vi "Main.vi"(11 "Module Admin":refnum<class "Delacor_lib_QMH_Cloneable Module Admin.lvclass">) -> ()   [LabVIEW 2020, in "Oscilloscope.lvlib"]
doc: "This template is based off of the Queued Message Handler design pattern and the Queued Message Handler project template that ships with LabVIEW.\n\nThe main difference is that the queue is private to this module and communication between modules is performed via Broadcast and Request events.\n\nRequest events are wrapped in public API methods and are handled in the Event Handling Loop (EHL) of this VI. Any module can register for Broadcast events sent by this module. The EHL generates messages based on user interface actions.\n\nThe Message Handling Loop (MHL) processes messages generated by the EHL, or by other messages. The messages are string values, so new messages can be added easily to the Message Cases case structure in the MHL. Each message cluster can also provide an optional value for Message Data, which is a variant that can be converted to whatever message-specific data is required.\n_____\nBased on DQMH Project Template 6.0.0.91."
uses:
  Oscilloscope.lvlib
  <vilib>/Delacor/Delacor QMH/Libraries/Cloneable Module Admin_class/Delacor_lib_QMH_Cloneable Module Admin.lvclass
  C:/Program Files (x86)/National Instruments/LabVIEW 2020/vi.lib/Delacor/Delacor QMH/Libraries/Module Admin_class/Delacor_lib_QMH_Module Admin.lvclass
  Module Data--cluster.ctl
  Clases/Osciloscopio/Osciloscopio.lvclass
  <vilib>/Delacor/Delacor QMH/Libraries/Message Queue_class/Delacor_lib_QMH_Message Queue.lvclass/Delacor_lib_QMH_Message Queue.ctl
  <vilib>/Delacor/Delacor QMH/Libraries/Cloneable Module Admin_class/Delacor_lib_QMH_Cloneable Module Admin.lvclass/Delacor_lib_QMH_Cloneable Module Admin.ctl
  Stop Argument--cluster.ctl
  <vilib>/Delacor/Delacor QMH/Libraries/Module Admin_class/Delacor_lib_QMH_Module Admin.lvclass/Delacor_lib_QMH_Module Admin.ctl
  Set COM Port Argument--cluster.ctl
  Initialize OSC Argument--cluster.ctl
  Close Argument--cluster.ctl
  Autosetup Argument--cluster.ctl
  Configure Channel Argument--cluster.ctl
  Read Waveform Argument--cluster.ctl
  Read Measurement Argument--cluster.ctl
  Read Measurement 2 Channels Argument--cluster.ctl
  Reset Argument--cluster.ctl
  <vilib>/Utility/miscctls.llb/LVPointTypeDef.ctl
  Clases/Osciloscopio/Osciloscopio.lvclass/Osciloscopio.ctl
  <vilib>/Delacor/Delacor QMH/Libraries/Message Queue_class/Delacor_lib_QMH_Enqueue Message (Single).vi
  <vilib>/Delacor/Delacor QMH/Libraries/Cloneable Module Admin_class/Delacor_lib_QMH_Get Module ID.vi
  <vilib>/Delacor/Delacor QMH/Libraries/Module Admin_class/Delacor_lib_QMH_Get External Launch.vi
  Clases/Osciloscopio/Write COM.vi
  <vilib>/Utility/error.llb/Error Cluster From Error Code.vi
  <vilib>/ErrorRing/Error Ring.xnode
  <vilib>/Delacor/Delacor QMH/Libraries/Message Queue_class/Delacor_lib_QMH_Message Queue.lvclass
panel:
  out "error out":errorcluster
  out "Status":string
  in  "Simulate EHL Error":bool
  in  "Simulate MHL Error":bool
  # "Other QMH Modules communicate with this Module via its Public API (wrappers for its Request Events).\n\nThis Module communicates with other Modules via its Broadcast Events.\nAny module that wants to get these messages, just registers for this module's Broadcast events."
  # "This template is for the Delacor Modified Queued Message Handler design pattern.\n\nSee the block diagram for more information on how to use this template."
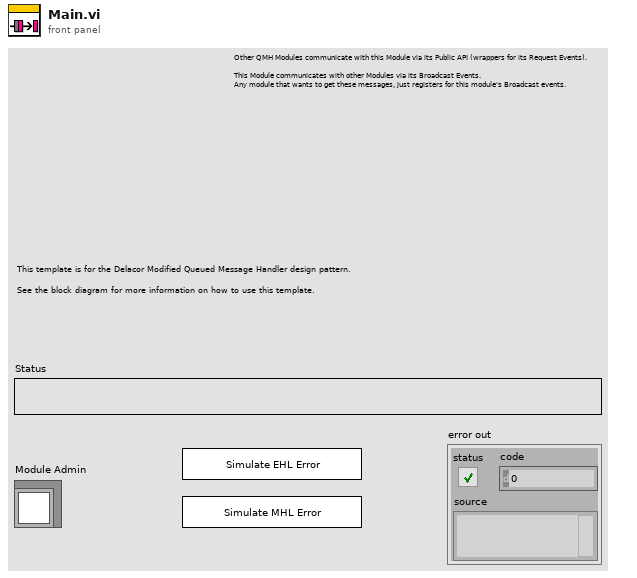
[diagram p1: front panel]
types:
  T1 = typedef "Oscilloscope.lvlib/Request Events--cluster.ctl" = cluster{"Stop Module":refnum<user-event>, "Show Panel":refnum<user-event>, "Hide Panel":refnum<user-event>, "Show Diagram":refnum<user-event>, "Get Module Execution Status":refnum<user-event>, "Set COM Port":refnum<user-event>, "Initialize OSC":refnum<user-event>, "Close":refnum<user-event>, "Autosetup":refnum<user-event>, "Configure Channel":refnum<user-event>, "Read Waveform":refnum<user-event>, "Read Measurement":refnum<user-event>, "Read Measurement 2 Channels":refnum<user-event>, "Reset":refnum<user-event>}
  T2 = typedef "Oscilloscope.lvlib/Module Data--cluster.ctl" = cluster{"Status":string, "Oscilloscope":refnum<class "Osciloscopio.lvclass">}
  T3 = enum32{"invalid lock state", "Not Locked", "Locked (No Password)", "Password-protected"}
  T4 = typedef "Oscilloscope.lvlib/Stop Argument--cluster.ctl" = cluster{"Module ID":i32, "Origin":string, "Exit via Stop Module Req?":bool, "Wait for Module to stop?":bool}
  T5 = typedef "Oscilloscope.lvlib/Set COM Port Argument--cluster.ctl" = cluster{"Module ID":i32, "COM":refnum<visa-resource-name>}
  T6 = typedef "Oscilloscope.lvlib/Initialize OSC Argument--cluster.ctl" = cluster{"Module ID":i32, "OSC Type":string}
  T7 = typedef "Oscilloscope.lvlib/Close Argument--cluster.ctl" = cluster{"Module ID":i32, "Boolean":bool}
  T8 = typedef "Oscilloscope.lvlib/Autosetup Argument--cluster.ctl" = cluster{"Module ID":i32, "Boolean":bool}
  T9 = typedef "Oscilloscope.lvlib/Configure Channel Argument--cluster.ctl" = cluster{"Module ID":i32, "Boolean":bool}
  T10 = typedef "Oscilloscope.lvlib/Read Waveform Argument--cluster.ctl" = cluster{"Module ID":i32, "Boolean":bool}
  T11 = typedef "Oscilloscope.lvlib/Read Measurement Argument--cluster.ctl" = cluster{"Module ID":i32, "Boolean":bool}
  T12 = typedef "Oscilloscope.lvlib/Read Measurement 2 Channels Argument--cluster.ctl" = cluster{"Module ID":i32, "Boolean":bool}
  T13 = typedef "Oscilloscope.lvlib/Reset Argument--cluster.ctl" = cluster{"Module ID":i32, "Boolean":bool}
  T14 = typedef "LVPointTypeDef.ctl" = cluster{"Horizontal":i16, "Vertical":i16}
  T15 = enum32{"Invalid", "Standard", "Closed", "Hidden", "Minimized", "Maximized"}
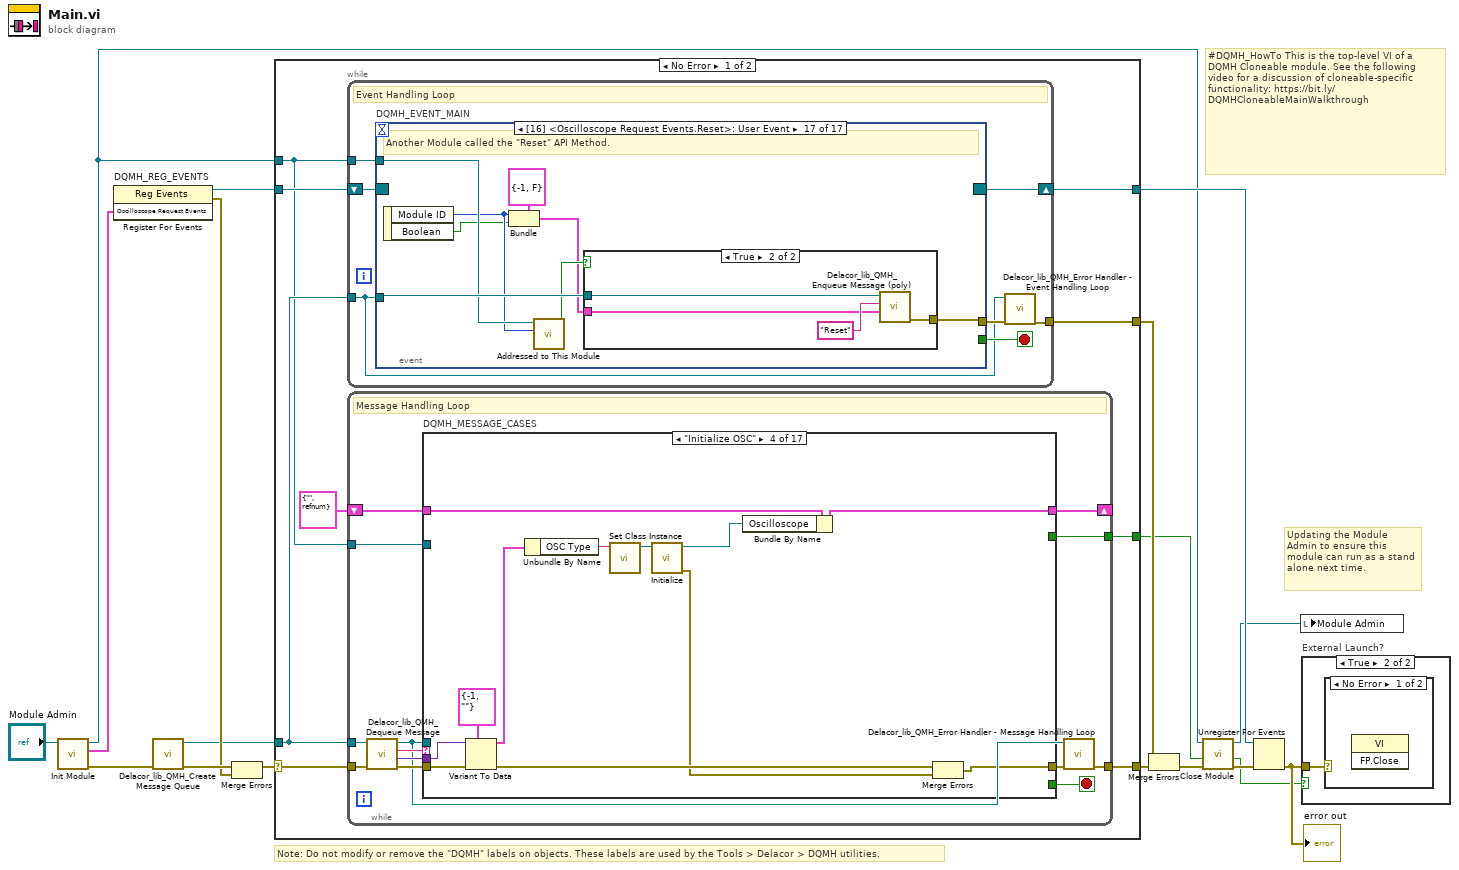
[diagram p0: block diagram]
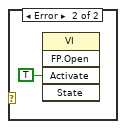
[diagram p3: hidden frame]
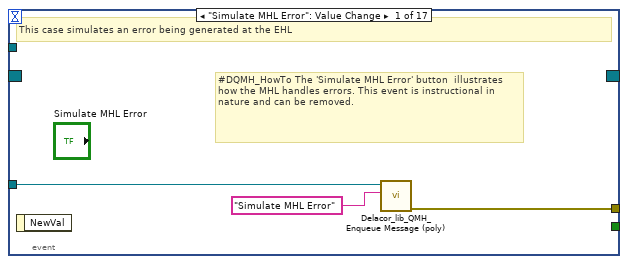
[diagram p4: hidden frame]
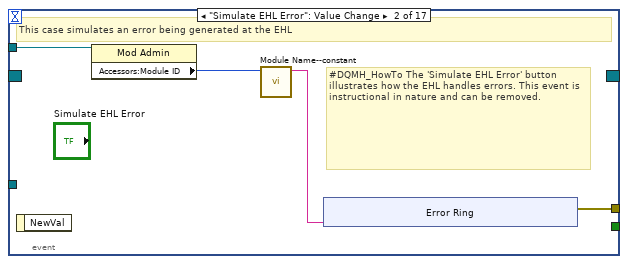
[diagram p5: hidden frame]
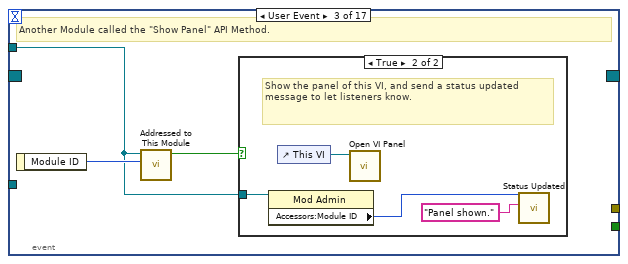
[diagram p6: hidden frame]
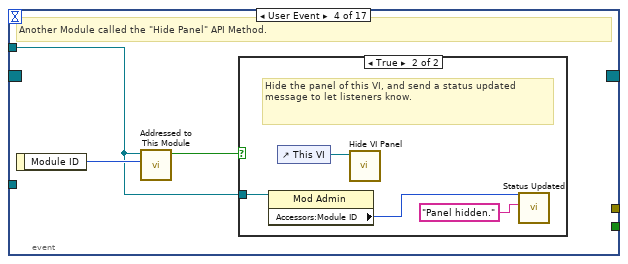
[diagram p8: hidden frame]
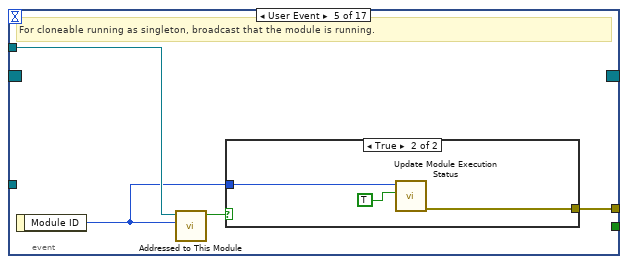
[diagram p10: hidden frame]
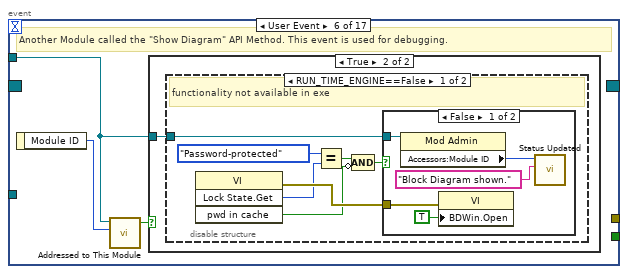
[diagram p12: hidden frame]
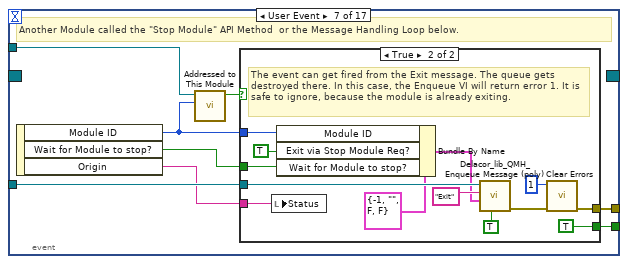
[diagram p16: hidden frame]
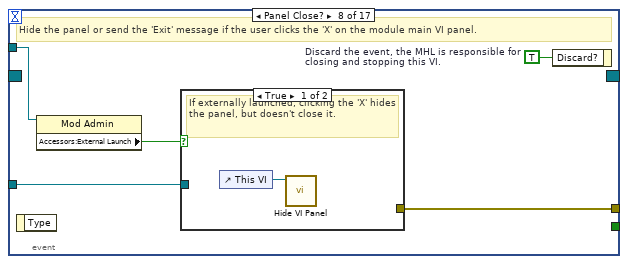
[diagram p18: hidden frame]
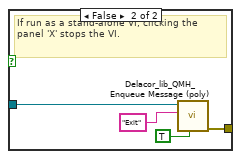
[diagram p19: hidden frame]
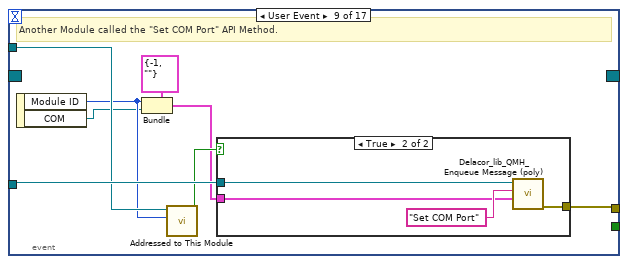
[diagram p20: hidden frame]
diagram:
  # "#DQMH_HowTo This is the top-level VI of a DQMH Cloneable module. See the following video for a discussion of cloneable-specific functionality: https://bit.ly/DQMHCloneableMainWalkthrough"
  # "Note: Do not modify or remove the \"DQMH\" labels on objects. These labels are used by the Tools > Delacor > DQMH utilities."
  # "Updating the Module Admin to ensure this module can run as a stand alone next time."
  n1 = call "Init Module.vi"("Cloneable Module Admin in"="Module Admin") -> ("error out"=w15:errorcluster, "Oscilloscope Request Events"=w7:T1, "Cloneable Module Admin out"=w4:refnum<class "Delacor_lib_QMH_Cloneable Module Admin.lvclass">)  [unwired: 8 in]
  n2 = register-events "DQMH_REG_EVENTS"(w7) -> (reference out=w8:refnum<event-registration>, error out=w10:errorcluster)  [unwired: 2 in]
  n3 = call <vilib>:"Delacor_lib_QMH_Create Message Queue.vi"("error in"=w15) -> ("error out"=w12:errorcluster, "Message Queue"=w6:refnum<class "Delacor_lib_QMH_Message Queue.lvclass">)  [unwired: 9 in]
  n4 = Merge Errors(w12, w10) -> (w11:errorcluster)
  n5 = case shown="No Error" w11 {
    selector: w11 -> [w25 w442]
    tunnel: [w27 w441] -> w16
    tunnel: [w24 w449] -> w9
    tunnel: w8 -> [w22 w449]
    tunnel: w6 -> [w21 w440]
    tunnel: [w26 _] -> w17
    tunnel: w4 -> [w20 w445]
    tunnel: [w19 _] -> w2
    frame No Error {
      n6 = while {
        tunnel: w21 -> [w28]
        shift-right: [w31] -> w24
        shift-left: w22 -> [w32]
        tunnel: [w33] -> w26
        tunnel: w20 -> [w29]
        stop <- w30 stop-if-true
        # "Event Handling Loop"
        n7 = event "DQMH_EVENT_MAIN" shown="[16] <Oscilloscope Request Events.Reset>: User Event" {
          selector: w32 -> [_ _ _ _ _ _ _ _ _ _ _ _ _ _ _ _ _]
          dyn-events: [_ _ _ _ _ _ _ _ _ _ _ _ _ _ _ _ _] -> w31
          timeout: _ -> [_ _ _ _ _ _ _ _ _ _ _ _ _ _ _ _ _]
          tunnel: [_ _ _ _ _ _ w89 _ _ _ _ _ _ _ _ _ _] -> w30
          tunnel: w28 -> [w36 _ _ _ _ _ w92 w108 w124 w136 w148 w160 w172 w184 w196 w208 w220]
          tunnel: [w37 w41 _ _ w66 _ w93 w111 w117 w129 w141 w153 w165 w177 w189 w201 w213] -> w34
          tunnel: w29 -> [_ w40 w49 w56 w64 w70 w91 w109 w122 w134 w146 w158 w170 w182 w194 w206 w218]
          event "Simulate MHL Error": Value Change {
            # "#DQMH_HowTo The 'Simulate MHL Error' button  illustrates how the MHL handles errors. This event is instructional in nature and can be removed."
            # "This case simulates an error being generated at the EHL"
            n8 = event-data() -> ()  [unwired: 1 in, 1 out]
            n9 = call-poly <vilib>:"Delacor_lib_QMH_Enqueue Message (poly).vi"("Message"="Simulate MHL Error", "Message Queue in"=w36) -> ("error out"=w37:errorcluster)  [unwired: 8 in, 1 out]
          }
          event "Simulate EHL Error": Value Change {
            # "#DQMH_HowTo The 'Simulate EHL Error' button  illustrates how the EHL handles errors. This event is instructional in nature and can be removed."
            # "This case simulates an error being generated at the EHL"
            n10 = event-data() -> ()  [unwired: 1 in, 1 out]
            n11 = property class="Mod Admin"(reference=w40) -> ("Accessors:Module ID"=w39:i32)  [unwired: 1 in, 2 out]
            n12 = call "Module Name--constant.vi"("Module ID"=w39) -> ("Module Name"=w38:string)  [unwired: 10 in]
            n13 = xnode "Error Ring"("parameter 0"=w38) -> ("error out"=w41:errorcluster)
          }
          event User Event {
            # "Another Module called the \"Show Panel\" API Method."
            n14 = event-data() -> ("Module ID"=w50:i32)  [unwired: 1 in]
            n15 = call "Addressed to This Module.vi"("Module ID from Argument"=w50, "Module Admin"=w49) -> ("Addressed to this instance?"=w51:bool)  [unwired: 8 in, 1 out]
            n16 = case shown="True" w51 {
              tunnel: w49 -> [_ w53]
              frame False {
              }
              frame True {
                # "Show the panel of this VI, and send a status updated message to let listeners know."
                n17 = property class="Mod Admin"(reference=w53) -> ("Accessors:Module ID"=w52:i32)  [unwired: 1 in, 2 out]
                n18 = control-ref of="This VI"() -> (w55:refnum<vi>)
                n19 = call "Open VI Panel.vi"("VI"=w55) -> ()  [unwired: 10 in, 1 out]
                n20 = call "Status Updated.vi"("Status"="Panel shown." ("format string"), "Module ID"=w52) -> ()  [unwired: 9 in, 1 out]
              }
            }
          }
          event User Event {
            # "Another Module called the \"Hide Panel\" API Method."
            n21 = event-data() -> ("Module ID"=w57:i32)  [unwired: 1 in]
            n22 = call "Addressed to This Module.vi"("Module ID from Argument"=w57, "Module Admin"=w56) -> ("Addressed to this instance?"=w58:bool)  [unwired: 8 in, 1 out]
            n23 = case shown="True" w58 {
              tunnel: w56 -> [_ w60]
              frame False {
              }
              frame True {
                # "Hide the panel of this VI, and send a status updated message to let listeners know."
                n24 = property class="Mod Admin"(reference=w60) -> ("Accessors:Module ID"=w59:i32)  [unwired: 1 in, 2 out]
                n25 = control-ref of="This VI"() -> (w62:refnum<vi>)
                n26 = call "Hide VI Panel.vi"("VI"=w62) -> ()  [unwired: 10 in, 1 out]
                n27 = call "Status Updated.vi"("Status"="Panel hidden." ("format string"), "Module ID"=w59) -> ()  [unwired: 9 in, 1 out]
              }
            }
          }
          event User Event {
            # "For cloneable running as singleton, broadcast that the module is running."
            n28 = event-data() -> ("Module ID"=w63:i32)  [unwired: 1 in]
            n29 = call "Addressed to This Module.vi"("Module ID from Argument"=w63, "Module Admin"=w64) -> ("Addressed to this instance?"=w65:bool)  [unwired: 8 in, 1 out]
            n30 = case shown="True" w65 {
              tunnel: [_ w69] -> w66
              tunnel: w63 -> [_ w68]
              frame False {
              }
              frame True {
                n31 = call "Update Module Execution Status.vi"("Running?"=TRUE, "Module ID"=w68) -> ("error out"=w69:errorcluster)  [unwired: 9 in]
              }
            }
          }
          event User Event {
            # "Another Module called the \"Show Diagram\" API Method. This event is used for debugging."
            n32 = event-data() -> ("Module ID"=w71:i32)  [unwired: 1 in]
            n33 = call "Addressed to This Module.vi"("Module ID from Argument"=w71, "Module Admin"=w70) -> ("Addressed to this instance?"=w72:bool)  [unwired: 8 in, 1 out]
            n34 = case shown="True" w72 {
              tunnel: w70 -> [_ w73]
              frame False {
              }
              frame True {
                n35 = disable-structure shown="RUN_TIME_ENGINE==False" {
                  disable-tunnel: w73 -> [w74 _]
                  frame condition #0 (active) {
                    # "functionality not available in exe"
                    n36 = invoke class="VI" method="Lock State.Get"() -> (error out=w80:errorcluster, "Get Lock State"=w79:T3, "pwd in cache"=w76:bool)  [unwired: 4 in, 1 out]
                    n37 = Equal?(x=T3."Password-protected", y=w79) -> (x = y?=w77:bool)
                    n38 = Compound Arithmetic op=AND(w77, invert w76) -> (w75:bool)
                    n39 = case shown="False" w75 {
                      tunnel: w80 -> [w85 _]
                      tunnel: w74 -> [w82 _]
                      frame False {
                        n40 = property class="Mod Admin"(reference=w82) -> ("Accessors:Module ID"=w81:i32)  [unwired: 1 in, 2 out]
                        n41 = property class="VI"(error in=w85, "BDWin.Open"=TRUE ("Block Diagram Window:Open")) -> ()  [unwired: 1 in, 2 out]
                        n42 = call "Status Updated.vi"("Status"="Block Diagram shown." ("format string"), "Module ID"=w81) -> ()  [unwired: 9 in, 1 out]
                      }
                      frame True {
                        # "Password-protected VI, and the password is not in the cache. Do not show the diagram."
                      }
                    }
                  }
                  frame condition #1 {
                  }
                }
              }
            }
          }
          event User Event {
            # "Another Module called the \"Stop Module\" API Method  or the Message Handling Loop below."
            n43 = event-data() -> ("Module ID"=w87:i32, "Wait for Module to stop?"=w88:bool, "Origin"=w86:string)  [unwired: 1 in]
            n44 = call "Addressed to This Module.vi"("Module ID from Argument"=w87, "Module Admin"=w91) -> ("Addressed to this instance?"=w90:bool)  [unwired: 8 in, 1 out]
            n45 = case shown="True" w90 {
              tunnel: [_ w105] -> w93
              tunnel: w92 -> [_ w101]
              tunnel: [_ TRUE] -> w89
              tunnel: w88 -> [_ w96]
              tunnel: w87 -> [_ w98]
              tunnel: w86 -> [_ w94]
              frame False {
              }
              frame True {
                # "The event can get fired from the Exit message. The queue gets destroyed there. In this case, the Enqueue VI will return error 1. It is safe to ignore, because the module is already exiting."
                n46 = local write "Status"(w94) -> ()
                n47 = Bundle By Name(cluster=T4 {"Module ID"=-1, "Origin"="", "Exit via Stop Module Req?"=FALSE, "Wait for Module to stop?"=FALSE} ("Stop Argument"), "Module ID"=w98, "Exit via Stop Module Req?"=TRUE, "Wait for Module to stop?"=w96) -> (w95:T4)
                n48 = call-poly <vilib>:"Delacor_lib_QMH_Enqueue Message (poly).vi"("Priority Message? (F)"=TRUE, "Message Data"=w95, "Message"="Exit", "Message Queue in"=w101) -> ("error out"=w106:errorcluster)  [unwired: 6 in, 1 out]
                n49 = call <vilib>:"Clear Errors.vi"("error in (no error)"=w106, "specific error code to clear (0: all)"=1) -> ("error out"=w105:errorcluster)  [unwired: 4 in, 1 out]
              }
            }
          }
          event Panel Close? {
            w110 = TRUE  # Discard the event, the MHL is responsible for closing and stopping this VI.
            # "Hide the panel or send the 'Exit' message if the user clicks the 'X' on the module main VI panel."
            n50 = event-data() -> ()  [unwired: 1 in, 1 out]
            n51 = property class="Mod Admin"(reference=w109) -> ("Accessors:External Launch"=w107:bool)  [unwired: 1 in, 2 out]
            n52 = case shown="True" w107 {
              tunnel: w108 -> [_ w115]
              tunnel: [_ w116] -> w111
              frame True {
                # "If externally launched, clicking the 'X' hides the panel, but doesn't close it."
                n53 = control-ref of="This VI"() -> (w112:refnum<vi>)
                n54 = call "Hide VI Panel.vi"("VI"=w112) -> ()  [unwired: 10 in, 1 out]
              }
              frame False {
                # "If run as a stand-alone VI, clicking the panel 'X' stops the VI."
                n55 = call-poly <vilib>:"Delacor_lib_QMH_Enqueue Message (poly).vi"("Priority Message? (F)"=TRUE, "Message"="Exit", "Message Queue in"=w115) -> ("error out"=w116:errorcluster)  [unwired: 7 in, 1 out]
              }
            }
            n56 = event-data("Discard?"=w110) -> ()  [unwired: 1 in, 1 out]
          }
          event User Event {
            # "Another Module called the \"Set COM Port\" API Method."
            n57 = event-data() -> ("Module ID"=w119:i32, "COM"=w118:refnum<visa-resource-name>)  [unwired: 1 in]
            n58 = Bundle(cluster=T5 {"Module ID"=-1, "COM"=""} ("Set COM Port Argument"), "Module ID"=w119, "COM"=w118) -> (w120:T5)
            n59 = call "Addressed to This Module.vi"("Module ID from Argument"=w119, "Module Admin"=w122) -> ("Addressed to this instance?"=w123:bool)  [unwired: 8 in, 1 out]
            n60 = case shown="True" w123 {
              tunnel: w124 -> [_ w128]
              tunnel: w120 -> [_ w126]
              tunnel: [_ w125] -> w117
              frame False {
              }
              frame True {
                n61 = call-poly <vilib>:"Delacor_lib_QMH_Enqueue Message (poly).vi"("Message Data"=w126, "Message"="Set COM Port", "Message Queue in"=w128) -> ("error out"=w125:errorcluster)  [unwired: 7 in, 1 out]
              }
            }
          }
          event User Event {
            # "Another Module called the \"Initialize OSC\" API Method."
            n62 = event-data() -> ("Module ID"=w131:i32, "OSC Type"=w130:string)  [unwired: 1 in]
            n63 = Bundle(cluster=T6 {"Module ID"=-1, "OSC Type"=""} ("Initialize OSC Argument"), "Module ID"=w131, "OSC Type"=w130) -> (w132:T6)
            n64 = call "Addressed to This Module.vi"("Module ID from Argument"=w131, "Module Admin"=w134) -> ("Addressed to this instance?"=w135:bool)  [unwired: 8 in, 1 out]
            n65 = case shown="True" w135 {
              tunnel: w136 -> [_ w140]
              tunnel: w132 -> [_ w138]
              tunnel: [_ w137] -> w129
              frame False {
              }
              frame True {
                n66 = call-poly <vilib>:"Delacor_lib_QMH_Enqueue Message (poly).vi"("Message Data"=w138, "Message"="Initialize OSC", "Message Queue in"=w140) -> ("error out"=w137:errorcluster)  [unwired: 7 in, 1 out]
              }
            }
          }
          event User Event {
            # "Another Module called the \"Close\" API Method."
            n67 = event-data() -> ("Module ID"=w143:i32, "Boolean"=w142:bool)  [unwired: 1 in]
            n68 = Bundle(cluster=T7 {"Module ID"=-1, "Boolean"=FALSE} ("Close Argument"), "Module ID"=w143, "Boolean"=w142) -> (w144:T7)
            n69 = call "Addressed to This Module.vi"("Module ID from Argument"=w143, "Module Admin"=w146) -> ("Addressed to this instance?"=w147:bool)  [unwired: 8 in, 1 out]
            n70 = case shown="True" w147 {
              tunnel: w148 -> [_ w152]
              tunnel: w144 -> [_ w150]
              tunnel: [_ w149] -> w141
              frame False {
              }
              frame True {
                n71 = call-poly <vilib>:"Delacor_lib_QMH_Enqueue Message (poly).vi"("Message Data"=w150, "Message"="Close", "Message Queue in"=w152) -> ("error out"=w149:errorcluster)  [unwired: 7 in, 1 out]
              }
            }
          }
          event User Event {
            # "Another Module called the \"Autosetup\" API Method."
            n72 = event-data() -> ("Module ID"=w155:i32, "Boolean"=w154:bool)  [unwired: 1 in]
            n73 = Bundle(cluster=T8 {"Module ID"=-1, "Boolean"=FALSE} ("Autosetup Argument"), "Module ID"=w155, "Boolean"=w154) -> (w156:T8)
            n74 = call "Addressed to This Module.vi"("Module ID from Argument"=w155, "Module Admin"=w158) -> ("Addressed to this instance?"=w159:bool)  [unwired: 8 in, 1 out]
            n75 = case shown="True" w159 {
              tunnel: w160 -> [_ w164]
              tunnel: w156 -> [_ w162]
              tunnel: [_ w161] -> w153
              frame False {
              }
              frame True {
                n76 = call-poly <vilib>:"Delacor_lib_QMH_Enqueue Message (poly).vi"("Message Data"=w162, "Message"="Autosetup", "Message Queue in"=w164) -> ("error out"=w161:errorcluster)  [unwired: 7 in, 1 out]
              }
            }
          }
          event User Event {
            # "Another Module called the \"Configure Channel\" API Method."
            n77 = event-data() -> ("Module ID"=w167:i32, "Boolean"=w166:bool)  [unwired: 1 in]
            n78 = Bundle(cluster=T9 {"Module ID"=-1, "Boolean"=FALSE} ("Configure Channel Argument"), "Module ID"=w167, "Boolean"=w166) -> (w168:T9)
            n79 = call "Addressed to This Module.vi"("Module ID from Argument"=w167, "Module Admin"=w170) -> ("Addressed to this instance?"=w171:bool)  [unwired: 8 in, 1 out]
            n80 = case shown="True" w171 {
              tunnel: w172 -> [_ w176]
              tunnel: w168 -> [_ w174]
              tunnel: [_ w173] -> w165
              frame False {
              }
              frame True {
                n81 = call-poly <vilib>:"Delacor_lib_QMH_Enqueue Message (poly).vi"("Message Data"=w174, "Message"="Configure Channel", "Message Queue in"=w176) -> ("error out"=w173:errorcluster)  [unwired: 7 in, 1 out]
              }
            }
          }
          event User Event {
            # "Another Module called the \"Read Waveform\" API Method."
            n82 = event-data() -> ("Module ID"=w179:i32, "Boolean"=w178:bool)  [unwired: 1 in]
            n83 = Bundle(cluster=T10 {"Module ID"=-1, "Boolean"=FALSE} ("Read Waveform Argument"), "Module ID"=w179, "Boolean"=w178) -> (w180:T10)
            n84 = call "Addressed to This Module.vi"("Module ID from Argument"=w179, "Module Admin"=w182) -> ("Addressed to this instance?"=w183:bool)  [unwired: 8 in, 1 out]
            n85 = case shown="True" w183 {
              tunnel: w184 -> [_ w188]
              tunnel: w180 -> [_ w186]
              tunnel: [_ w185] -> w177
              frame False {
              }
              frame True {
                n86 = call-poly <vilib>:"Delacor_lib_QMH_Enqueue Message (poly).vi"("Message Data"=w186, "Message"="Read Waveform", "Message Queue in"=w188) -> ("error out"=w185:errorcluster)  [unwired: 7 in, 1 out]
              }
            }
          }
          event User Event {
            # "Another Module called the \"Read Measurement\" API Method."
            n87 = event-data() -> ("Module ID"=w191:i32, "Boolean"=w190:bool)  [unwired: 1 in]
            n88 = Bundle(cluster=T11 {"Module ID"=-1, "Boolean"=FALSE} ("Read Measurement Argument"), "Module ID"=w191, "Boolean"=w190) -> (w192:T11)
            n89 = call "Addressed to This Module.vi"("Module ID from Argument"=w191, "Module Admin"=w194) -> ("Addressed to this instance?"=w195:bool)  [unwired: 8 in, 1 out]
            n90 = case shown="True" w195 {
              tunnel: w196 -> [_ w200]
              tunnel: w192 -> [_ w198]
              tunnel: [_ w197] -> w189
              frame False {
              }
              frame True {
                n91 = call-poly <vilib>:"Delacor_lib_QMH_Enqueue Message (poly).vi"("Message Data"=w198, "Message"="Read Measurement", "Message Queue in"=w200) -> ("error out"=w197:errorcluster)  [unwired: 7 in, 1 out]
              }
            }
          }
          event User Event {
            # "Another Module called the \"Read Measurement 2 Channels\" API Method."
            n92 = event-data() -> ("Module ID"=w203:i32, "Boolean"=w202:bool)  [unwired: 1 in]
            n93 = Bundle(cluster=T12 {"Module ID"=-1, "Boolean"=FALSE} ("Read Measurement 2 Channels Argument"), "Module ID"=w203, "Boolean"=w202) -> (w204:T12)
            n94 = call "Addressed to This Module.vi"("Module ID from Argument"=w203, "Module Admin"=w206) -> ("Addressed to this instance?"=w207:bool)  [unwired: 8 in, 1 out]
            n95 = case shown="True" w207 {
              tunnel: w208 -> [_ w212]
              tunnel: w204 -> [_ w210]
              tunnel: [_ w209] -> w201
              frame False {
              }
              frame True {
                n96 = call-poly <vilib>:"Delacor_lib_QMH_Enqueue Message (poly).vi"("Message Data"=w210, "Message"="Read Measurement 2 Channels", "Message Queue in"=w212) -> ("error out"=w209:errorcluster)  [unwired: 7 in, 1 out]
              }
            }
          }
          event User Event {
            # "Another Module called the \"Reset\" API Method."
            n97 = event-data() -> ("Module ID"=w215:i32, "Boolean"=w214:bool)  [unwired: 1 in]
            n98 = Bundle(cluster=T13 {"Module ID"=-1, "Boolean"=FALSE} ("Reset Argument"), "Module ID"=w215, "Boolean"=w214) -> (w216:T13)
            n99 = call "Addressed to This Module.vi"("Module ID from Argument"=w215, "Module Admin"=w218) -> ("Addressed to this instance?"=w219:bool)  [unwired: 8 in, 1 out]
            n100 = case shown="True" w219 {
              tunnel: w220 -> [_ w224]
              tunnel: w216 -> [_ w222]
              tunnel: [_ w221] -> w213
              frame False {
              }
              frame True {
                n101 = call-poly <vilib>:"Delacor_lib_QMH_Enqueue Message (poly).vi"("Message Data"=w222, "Message"="Reset", "Message Queue in"=w224) -> ("error out"=w221:errorcluster)  [unwired: 7 in, 1 out]
              }
            }
          }
        }
        n102 = call-dynamic "Delacor_lib_QMH_Error Handler - Event Handling Loop.vi"("error in"=w34, "Message Queue in"=w28) -> ("dup error in"=w33:errorcluster)  [unwired: 8 in, 1 out]
      }
      n103 = while {
        tunnel: w21 -> [w228]
        shift-right: [w232] -> _
        shift-left: T2 {"Status"="", "Oscilloscope"=refnum} ("Data Cluster") -> [w233]
        tunnel: w25 -> [w236]
        tunnel: [w234] -> w27
        tunnel: w20 -> [w226]
        tunnel: [w225] -> w19
        stop <- w231 stop-if-true
        # "Message Handling Loop"
        n104 = call-dynamic "Delacor_lib_QMH_Dequeue Message.vi"("error in"=w236, "Message Queue in"=w228) -> ("error out"=w235:errorcluster, "Message Data"=w229:variant, "Message"=w230:string, "Message Queue out"=w227:refnum<class "Delacor_lib_QMH_Message Queue.lvclass">)  [unwired: 6 in]
        n105 = case "DQMH_MESSAGE_CASES" shown="\"Initialize OSC\"" w230 {
          selector: w230 -> [_ _ _ _ _ _ _ _ _ _ _ _ _ _ _ _ w427]
          tunnel: w227 -> [_ _ _ _ _ _ _ _ _ _ _ _ _ w378 _ w417 _]
          tunnel: w235 -> [w257 w261 w271 w287 w296 w308 w320 w332 w344 w356 w368 w374 w376 w387 w400 w423 w429]
          tunnel: [w255 w261 w263 w280 w289 w301 w313 w325 w337 w349 w361 w373 w376 w383 w399 w420 w430] -> w237
          tunnel: w233 -> [w248 w260 w266 w282 w291 w303 w315 w327 w339 w351 w363 w372 w375 w382 w397 w416 w428]
          tunnel: [w247 w260 w265 w281 w290 w302 w314 w326 w338 w350 w362 w372 w375 w382 w397 w416 w428] -> w232
          tunnel: [_ _ _ _ _ _ _ _ _ _ _ _ _ _ _ w415 _] -> w231
          tunnel: w229 -> [_ _ w269 w285 w294 w306 w318 w330 w342 w354 w366 _ _ w381 _ w413 _]
          tunnel: w226 -> [w243 _ _ _ _ _ _ _ _ _ _ _ _ w380 w395 w409 w425]
          tunnel: [_ _ _ _ _ _ _ _ _ _ _ _ _ _ _ w411 _] -> w225
          frame "Initialize" {
            w240 = "Initial Message" ("Initial Message")
            # "Initialize - Any operation that needs to be done before the module can receive messages. Synchronize Caller Events.vi will inform Start Module.vi that the module has launched and is ready to receive messages. Module Did Init.vi will broadcast that the module initialized."
            n106 = call "Synchronize Caller Events.vi"("error in (no error)"=w257, "Module Admin"=w243) -> ("error out"=w256:errorcluster, "Module Admin out"=w242:refnum<class "Delacor_lib_QMH_Cloneable Module Admin.lvclass">)  [unwired: 8 in]
            n107 = call "Get Classes Names.vi"() -> ("Array"=w239:string[])  [unwired: 11 in]
            n108 = property class="Mod Admin"(reference=w242) -> ("Accessors:Module ID"=w238:i32, "Accessors:External Launch"=w244:bool)  [unwired: 1 in, 2 out]
            n109 = call "OSC Availables.vi"("OSC Type"=w239, "Module ID"=w238) -> ()  [unwired: 9 in, 1 out]
            n110 = call "Module Name--constant.vi"("Module ID"=w238) -> ("Module Name"=w252:string)  [unwired: 10 in]
            n111 = property class="VI"("Front Panel.Title"=w252) -> (reference out=w254:refnum<vi>, error out=w259:errorcluster)  [unwired: 2 in]
            n112 = Select(t=T15."Hidden" ("State"), s=w244, f=T15."Standard" ("State")) -> (s? t:f=w249:T15)
            n113 = invoke class="VI" method="FP.Open"(reference=w254, error in=w259, "State"=w249) -> (reference out=w253:refnum<vi>, error out=w258:errorcluster)  [unwired: 2 in, 3 out]
            n114 = call "Module Name--constant.vi"("Module ID"=w238) -> ("Module Name"=w245:string)  [unwired: 10 in]
            n115 = Bundle By Name(cluster=w248, "Status"=w240) -> (w247:T2)
            n116 = invoke class="VI" method="FP.Center"(reference=w253, error in=w258) -> ()  [unwired: 1 in, 3 out]
            n117 = property on="Pane" class="Pane"("Origin"=T14 {"Horizontal"=0, "Vertical"=0}) -> ()  [unwired: 2 in, 2 out]
            n118 = call "Module Did Init.vi"("error in (no error)"=w256, "Initialized?"=TRUE, "Origin"=w245, "Module ID"=w238) -> ("error out"=w255:errorcluster)  [unwired: 7 in]
            "Status" <- w240
          }
          frame "---Module Specific---" {
            # "Separator -- The following cases handle messages specific to this Module."
          }
          frame "Set COM Port" {
            # "Set the COM Port"
            n119 = Variant To Data(error in=w271, type=T5 {"Module ID"=-1, "COM"=""} ("Set COM Port Argument"), Variant=w269) -> (data=w267:T5, error out=w270:errorcluster)
            n120 = Unbundle By Name(w267) -> ("COM"=w264:refnum<visa-resource-name>)
            n121 = in-place {
              in-place-border: w264 -> [w275]
              in-place-border: [w272] -> w262
              n122 = in-place-cluster #1(w266) -> ("Oscilloscope"=w274:refnum<class "Osciloscopio.lvclass">)
              n123 = property class="Osciloscopio.lvclass"(reference=w274, "Accessors:COM"=w275) -> (reference out=w273:refnum<class "Osciloscopio.lvclass">, error out=w272:errorcluster)  [unwired: 1 in]
              n124 = in-place-cluster #1("Oscilloscope"=w273) -> (w265:T2)
            }
            n125 = Merge Errors(w270, w262) -> (w263:errorcluster)
          }
          frame "Initialize OSC" {
            n126 = Variant To Data(error in=w287, type=T6 {"Module ID"=-1, "OSC Type"=""} ("Initialize OSC Argument"), Variant=w285) -> (data=w283:T6, error out=w286:errorcluster)
            n127 = Unbundle By Name(w283) -> ("OSC Type"=w278:string)
            n128 = call "Set Class Instance.vi"("OSC Type"=w278) -> ("element"=w276:refnum<class "Osciloscopio.lvclass">)  [unwired: 10 in]
            n129 = call-dynamic "Initialize.vi"("Osciloscopio in"=w276) -> ("error out"=w279:errorcluster, "Osciloscopio out"=w277:refnum<class "Osciloscopio.lvclass">)  [unwired: 9 in]
            n130 = Bundle By Name(cluster=w282, "Oscilloscope"=w277) -> (w281:T2)
            n131 = Merge Errors(w286, w279) -> (w280:errorcluster)
          }
          frame "Close" {
            # "Close OSC"
            n132 = Variant To Data(error in=w296, type=T7 {"Module ID"=-1, "Boolean"=FALSE} ("Close Argument"), Variant=w294) -> (data=w292:T7, error out=w295:errorcluster)
            n133 = Unbundle By Name(w292) -> ()  [unwired: 2 out]
            n134 = in-place {
              in-place-border: [w297] -> w288
              n135 = in-place-cluster #2(w291) -> ("Oscilloscope"=w299:refnum<class "Osciloscopio.lvclass">)
              n136 = call-dynamic "Close.vi"("Osciloscopio in"=w299) -> ("error out"=w297:errorcluster, "Osciloscopio out"=w298:refnum<class "Osciloscopio.lvclass">)  [unwired: 9 in]
              n137 = in-place-cluster #2("Oscilloscope"=w298) -> (w290:T2)
            }
            n138 = Merge Errors(w295, w288) -> (w289:errorcluster)
          }
          frame "Autosetup" {
            # "Autoset OSC"
            n139 = Variant To Data(error in=w308, type=T8 {"Module ID"=-1, "Boolean"=FALSE} ("Autosetup Argument"), Variant=w306) -> (data=w304:T8, error out=w307:errorcluster)
            n140 = Unbundle By Name(w304) -> ()  [unwired: 2 out]
            n141 = in-place {
              in-place-border: [w309] -> w300
              n142 = in-place-cluster #3(w303) -> ("Oscilloscope"=w311:refnum<class "Osciloscopio.lvclass">)
              n143 = call-dynamic "Autosetup.vi"("Osciloscopio in"=w311) -> ("error out"=w309:errorcluster, "Osciloscopio out"=w310:refnum<class "Osciloscopio.lvclass">)  [unwired: 9 in]
              n144 = in-place-cluster #3("Oscilloscope"=w310) -> (w302:T2)
            }
            n145 = Merge Errors(w307, w300) -> (w301:errorcluster)
          }
          frame "Configure Channel" {
            # "Configure channel of OSC"
            n146 = Variant To Data(error in=w320, type=T9 {"Module ID"=-1, "Boolean"=FALSE} ("Configure Channel Argument"), Variant=w318) -> (data=w316:T9, error out=w319:errorcluster)
            n147 = Unbundle By Name(w316) -> ()  [unwired: 2 out]
            n148 = in-place {
              in-place-border: [w321] -> w312
              n149 = in-place-cluster #4(w315) -> ("Oscilloscope"=w323:refnum<class "Osciloscopio.lvclass">)
              n150 = call-dynamic "Configure Channel.vi"("Osciloscopio in"=w323) -> ("error out"=w321:errorcluster, "Osciloscopio out"=w322:refnum<class "Osciloscopio.lvclass">)  [unwired: 9 in]
              n151 = in-place-cluster #4("Oscilloscope"=w322) -> (w314:T2)
            }
            n152 = Merge Errors(w319, w312) -> (w313:errorcluster)
          }
          frame "Read Waveform" {
            # "Reads the waveform"
            n153 = Variant To Data(error in=w332, type=T10 {"Module ID"=-1, "Boolean"=FALSE} ("Read Waveform Argument"), Variant=w330) -> (data=w328:T10, error out=w331:errorcluster)
            n154 = in-place {
              in-place-border: [w333] -> w324
              n155 = in-place-cluster #5(w327) -> ("Oscilloscope"=w335:refnum<class "Osciloscopio.lvclass">)
              n156 = call-dynamic "Read (Waveform).vi"("Osciloscopio in"=w335) -> ("error out"=w333:errorcluster, "Osciloscopio out"=w334:refnum<class "Osciloscopio.lvclass">)  [unwired: 8 in, 1 out]
              n157 = in-place-cluster #5("Oscilloscope"=w334) -> (w326:T2)
            }
            n158 = Unbundle By Name(w328) -> ()  [unwired: 2 out]
            n159 = Merge Errors(w331, w324) -> (w325:errorcluster)
          }
          frame "Read Measurement" {
            # "Reads the measure"
            n160 = Variant To Data(error in=w344, type=T11 {"Module ID"=-1, "Boolean"=FALSE} ("Read Measurement Argument"), Variant=w342) -> (data=w340:T11, error out=w343:errorcluster)
            n161 = in-place {
              in-place-border: [w345] -> w336
              n162 = in-place-cluster #6(w339) -> ("Oscilloscope"=w347:refnum<class "Osciloscopio.lvclass">)
              n163 = call-dynamic "Read Measurement.vi"("Osciloscopio in"=w347) -> ("error out"=w345:errorcluster, "Osciloscopio out"=w346:refnum<class "Osciloscopio.lvclass">)  [unwired: 7 in, 2 out]
              n164 = in-place-cluster #6("Oscilloscope"=w346) -> (w338:T2)
            }
            n165 = Unbundle By Name(w340) -> ()  [unwired: 2 out]
            n166 = Merge Errors(w343, w336) -> (w337:errorcluster)
          }
          frame "Read Measurement 2 Channels" {
            # "Reads the measure of the 2 Channels of OSC"
            n167 = Variant To Data(error in=w356, type=T12 {"Module ID"=-1, "Boolean"=FALSE} ("Read Measurement 2 Channels Argument"), Variant=w354) -> (data=w352:T12, error out=w355:errorcluster)
            n168 = Unbundle By Name(w352) -> ()  [unwired: 2 out]
            n169 = in-place {
              in-place-border: [w357] -> w348
              n170 = in-place-cluster #7(w351) -> ("Oscilloscope"=w359:refnum<class "Osciloscopio.lvclass">)
              n171 = call-dynamic "Read Measurement 2 Channels.vi"("Osciloscopio in"=w359) -> ("error out"=w357:errorcluster, "Osciloscopio out"=w358:refnum<class "Osciloscopio.lvclass">)  [unwired: 7 in, 2 out]
              n172 = in-place-cluster #7("Oscilloscope"=w358) -> (w350:T2)
            }
            n173 = Merge Errors(w355, w348) -> (w349:errorcluster)
          }
          frame "Reset" {
            # "Resets the OSC"
            n174 = Variant To Data(error in=w368, type=T13 {"Module ID"=-1, "Boolean"=FALSE} ("Reset Argument"), Variant=w366) -> (data=w364:T13, error out=w367:errorcluster)
            n175 = in-place {
              in-place-border: [w369] -> w360
              n176 = in-place-cluster #8(w363) -> ("Oscilloscope"=w370:refnum<class "Osciloscopio.lvclass">)
              n177 = call-dynamic "Reset.vi"("Osciloscopio in"=w370) -> ("error out"=w369:errorcluster, "Osciloscopio out"=w371:refnum<class "Osciloscopio.lvclass">)  [unwired: 9 in]
              n178 = in-place-cluster #8("Oscilloscope"=w371) -> (w362:T2)
            }
            n179 = Unbundle By Name(w364) -> ()  [unwired: 2 out]
            n180 = Merge Errors(w367, w360) -> (w361:errorcluster)
          }
          frame "---Copy This Frame---" {
            # "Duplicate this frame when creating new messages.  Change this comment in the duplicated frame to describe this message."
            n181 = Merge Errors(w374) -> (w373:errorcluster)
          }
          frame "---Exit and Error Handling---" {
            # "Separator - the following cases handle errors and exit messages."
          }
          frame "Error" {
            # "#CodeRecommended - If you ever change the name of this \"Error\" message, you'll need to update the name in the Check Loop Error.vi as well."
            # "#CodeRecommended - If the module is running in standalone mode (External Launch = FALSE), this code will pop up an error dialog and call the 'Exit' message if an error occurs. Add more fine-grained error handling here."
            # "Error - Check the error message data and respond accordingly. This message is sent by the \"Error Handler\" VIs at the end of each loop in this application."
            n182 = property class="Mod Admin"(reference=w380) -> ("Accessors:External Launch"=w379:bool, "Accessors:Module ID"=w377:i32)  [unwired: 1 in, 2 out]
            n183 = Variant To Data(error in=w387, type=errorcluster {"status"=FALSE, "code"=0, "source"=""} ("error constant"), Variant=w381) -> (data=w388:errorcluster, error out=w385:errorcluster)
            n184 = call "Error Reported.vi"("Error"=w388, "Module ID"=w377) -> ()  [unwired: 9 in, 1 out]
            n185 = case shown="False" w379 {
              tunnel: [w393 _] -> w384
              tunnel: w378 -> [w391 _]
              tunnel: w388 -> [w392 _]
              frame False {
                # "If the module is running standalone, then pop up an error dialog and call the \"Exit\" message."
                n186 = call <vilib>:"Simple Error Handler.vi"("error in (no error)"=w392) -> ()  [unwired: 4 in, 5 out]
                n187 = call-poly <vilib>:"Delacor_lib_QMH_Enqueue Message (poly).vi"("Priority Message? (F)"=TRUE, "Message"="Exit", "Message Queue in"=w391) -> ("error out"=w393:errorcluster)  [unwired: 7 in, 1 out]
              }
              frame True {
                # "If the module was launched externally, calling the Error Reported broadcast VI is the only action performed by the \"Error\" message. The module's caller can then process the error appropriately."
              }
            }
            n188 = Merge Errors(w385, w384) -> (w383:errorcluster)
            n189 = local write "error out"(w383) -> ()
          }
          frame "Simulate MHL Error" {
            # "#DQMH_HowTo The 'Simulate MHL Error' button  illustrates how the MHL handles errors. This event is instructional in nature and can be removed."
            # "Simulate an error occurring at the MHL"
            n190 = property class="Mod Admin"(reference=w395) -> ("Accessors:Module ID"=w396:i32)  [unwired: 1 in, 2 out]
            n191 = call "Module Name--constant.vi"("Module ID"=w396) -> ("Module Name"=w394:string)  [unwired: 10 in]
            n192 = xnode "Error Ring"("parameter 0"=w394) -> ("error out"=w398:errorcluster)
            n193 = Merge Errors(w400, w398) -> (w399:errorcluster)
          }
          frame "Exit" {
            w414 = 91  # 91: not all Exit messages will have an argument
            w415 = TRUE  # Stop the VI
            # "Release the message queue reference"
            # "#CodeNeeded - Add any required cleanup code here."
            # "Exit - Exit the application."
            n194 = Variant To Data(error in=w423, type=T4 {"Module ID"=-1, "Origin"="", "Exit via Stop Module Req?"=FALSE, "Wait for Module to stop?"=FALSE} ("Stop Argument"), Variant=w413) -> (data=w410:T4, error out=w418:errorcluster)
            n195 = call <vilib>:"Clear Errors.vi"("error in (no error)"=w418, "specific error code to clear (0: all)"=w414) -> ("error out"=w422:errorcluster)  [unwired: 4 in, 1 out]
            n196 = control-ref of="This VI"() -> (w408:refnum<vi>)
            n197 = call-dynamic "Delacor_lib_QMH_Release Message Queue.vi"("error in"=w422, "Message Queue"=w417) -> ("error out"=w421:errorcluster)  [unwired: 9 in]
            n198 = call "Handle Exit.vi"("Stop Argument"=w410, "Module Admin in"=w409, "VI reference"=w408) -> ("error out"=w419:errorcluster, "Wait for Stop?"=w411:bool)  [unwired: 7 in]
            n199 = Merge Errors(w421, w419) -> (w420:errorcluster)
          }
          frame Default {
            # "'Default' case only runs if there is a message that isn't defined in any of the other cases.  Output a programming error."
            n200 = property class="Mod Admin"(reference=w425) -> ("Accessors:Module ID"=w424:i32)  [unwired: 1 in, 2 out]
            n201 = call "Module Name--constant.vi"("Module ID"=w424) -> ("Module Name"=w426:string)  [unwired: 10 in]
            n202 = xnode "Error Ring"("parameter 0"=w427, "parameter 1"=w426) -> ("error out"=w431:errorcluster)
            n203 = Merge Errors(w429, w431) -> (w430:errorcluster)
          }
        }
        n204 = call-dynamic "Delacor_lib_QMH_Error Handler - Message Handling Loop.vi"("error in"=w237, "Message Queue in"=w227) -> ("dup error in"=w234:errorcluster)  [unwired: 8 in, 1 out]
      }
    }
    frame Error {
      n205 = call "Synchronize Caller Events.vi"("Module Admin"=w445) -> ("Module Admin out"=w444:refnum<class "Delacor_lib_QMH_Cloneable Module Admin.lvclass">)  [unwired: 9 in, 1 out]
      n206 = property class="Mod Admin"(reference=w444) -> ("Accessors:Module ID"=w443:i32)  [unwired: 1 in, 2 out]
      n207 = call-dynamic "Delacor_lib_QMH_Release Message Queue.vi"("error in"=w442, "Message Queue"=w440) -> ("error out"=w441:errorcluster)  [unwired: 9 in]
      n208 = call "Module Name--constant.vi"("Module ID"=w443) -> ("Module Name"=w448:string)  [unwired: 10 in]
      n209 = Format Into String(format string="An error occurred during initialization. %s is no longer running.", w448) -> (resulting string=w446:string)  [unwired: 2 in, 1 out]
      n210 = call "Error Reported.vi"("Additional Information"=w446, "Error"=w441, "Module ID"=w443) -> ()  [unwired: 8 in, 1 out]
    }
  }
  n211 = Merge Errors(w17, w16) -> (w18:errorcluster)
  n212 = call "Close Module.vi"("error in"=w18, "Wait for stop?"=w2, "Module Admin in"=w4) -> ("error out"=w14:errorcluster, "External Launch"=w1:bool, "Module Admin out"=w3:refnum<class "Delacor_lib_QMH_Cloneable Module Admin.lvclass">)  [unwired: 6 in]
  n213 = Unregister For Events(event registration refnum=w9, error in=w14) -> (error out=w13:errorcluster)
  "error out" <- w13
  n214 = local write "Module Admin"(w3) -> ()
  n215 = case "External Launch?" shown="True" w1 {
    tunnel: w13 -> [_ w450]
    frame False {
    }
    frame True {
      n216 = case shown="No Error" w450 {
        frame No Error {
          n217 = invoke class="VI" method="FP.Close"() -> ()  [unwired: 3 in, 3 out]
        }
        frame Error {
          n218 = invoke class="VI" method="FP.Open"("Activate"=TRUE ("Activate?")) -> ()  [unwired: 4 in, 5 out]
        }
      }
    }
  }
